vi "HTTPS Server Test with TCPIP Nodes.vi"() -> ()   [LabVIEW 2013]
uses:
  NI OpenSSL Socket/SSL_Lib/SSL-Lib/Library Paths.ctl
  NI OpenSSL Socket/SSL_Lib/SSL/SSL_Mode.ctl
  NI OpenSSL Socket/SSL_Lib/SSL-Lib/SSL-Lib.lvclass
  NI OpenSSL Socket/SSL_Lib/SSL-Context/SSL-Context.lvclass
  NI OpenSSL Socket/SSL_Lib/SSL/SSL.lvclass
panel:
  in  "stop":bool
  out "Read bytes":string
  out "Numeric":i32
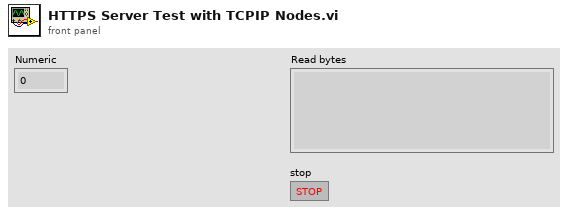
[diagram p1: front panel]
types:
  T1 = typedef "OpenSSL Socket.lvlib/SSL.lvclass/SSL_Mode.ctl" = i32
  T2 = typedef "OpenSSL Socket.lvlib/SSL-Lib.lvclass/Library Paths.ctl" = cluster{"SSL Library Path":path, "Crypto Library Path":path}
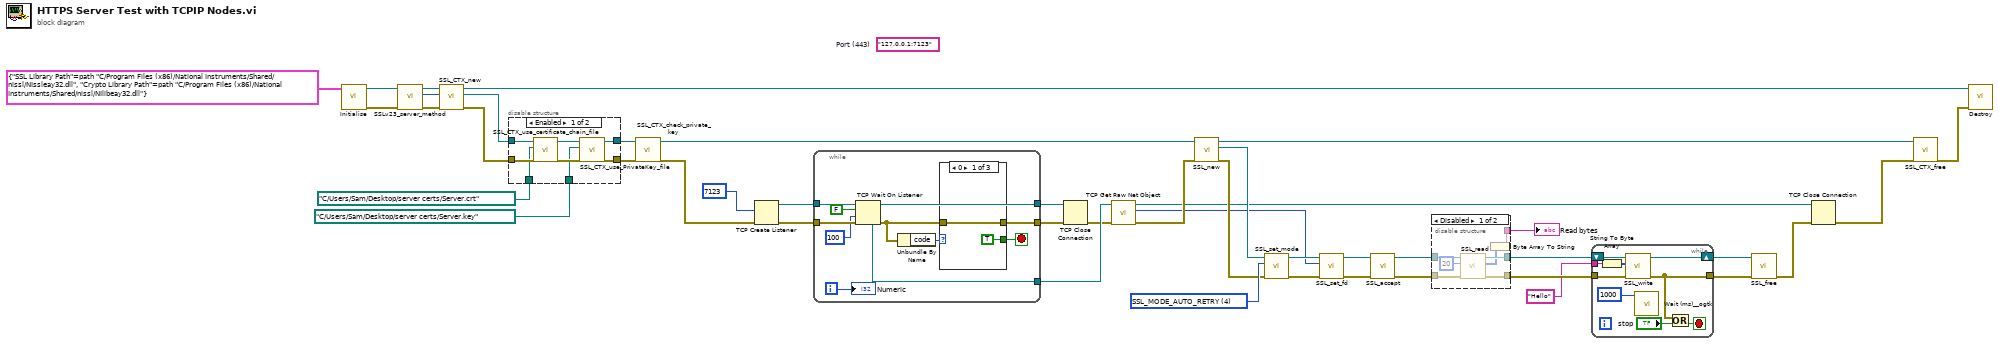
[diagram p0: block diagram]
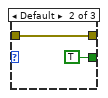
[diagram p3: hidden frame]
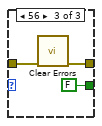
[diagram p4: hidden frame]
diagram:
  (unwired) "127.0.0.1:7123"  # Port (443)
  w31 = T1 4 items=["None"=0, "SSL_MODE_ENABLE_PARTIAL_WRITE"=1, "SSL_MODE_ACCEPT_MOVING_WRITE_BUFFER"=2, "SSL_MODE_AUTO_RETRY"=4, "SSL_MODE_RELEASE_BUFFERS"=16, "SSL_MODE_SEND_FALLBACK_SCSV"=128] ("Mode")
  n1 = call "Initialise.vi"("Library Paths"=T2 {"SSL Library Path"=path "C:/Program Files (x86)/National Instruments/Shared/nissl/NIssleay32.dll", "Crypto Library Path"=path "C:/Program Files (x86)/National Instruments/Shared/nissl/NIlibeay32.dll"}) -> ("error out"=w40:errorcluster, "SSL-Lib out"=w44:refnum<class "SSL-Lib.lvclass">)  [unwired: 9 in]
  n2 = call "SSLv23_server_method.vi"("error in (no error)"=w40, "SSL-Lib in"=w44) -> ("error out"=w38:errorcluster, "*SSL_Method"=w43:u64, "SSL-Lib out"=w42:refnum<class "SSL-Lib.lvclass">)  [unwired: 7 in]
  n3 = call "SSL_CTX_new.vi"("error in (no error)"=w38, "*SSL_Method"=w43, "SSL-Lib in"=w42) -> ("error out"=w37:errorcluster, "SSL-Context out"=w36:refnum<class "SSL-Context.lvclass">, "SSL-Lib out"=w30:refnum<class "SSL-Lib.lvclass">)  [unwired: 6 in]
  n4 = disable-structure shown="Enabled" {
    disable-tunnel: w37 -> [w50 w53]
    disable-tunnel: w36 -> [w49 w54]
    disable-tunnel: [w48 w53] -> w35
    disable-tunnel: [w47 w54] -> w34
    disable-tunnel: path "C:/Users/Sam/Desktop/server certs/Server.crt" -> [w46 _]
    disable-tunnel: path "C:/Users/Sam/Desktop/server certs/Server.key" -> [w45 _]
    frame Enabled {
      n5 = call "SSL_CTX_use_certificate_chain_file.vi"("error in (no error)"=w50, "Certificate Chain File"=w46, "SSL-Context in"=w49) -> ("error out"=w52:errorcluster, "SSL-Context out"=w51:refnum<class "SSL-Context.lvclass">)  [unwired: 7 in]
      n6 = call "SSL_CTX_use_PrivateKey_file.vi"("error in (no error)"=w52, "PrivateKey File"=w45, "SSL-Context in"=w51) -> ("error out"=w48:errorcluster, "SSL-Context out"=w47:refnum<class "SSL-Context.lvclass">)  [unwired: 7 in]
    }
    frame Disabled {
    }
  }
  n7 = call "SSL_CTX_check_private_key.vi"("error in (no error)"=w35, "SSL-Context in"=w34) -> ("error out"=w21:errorcluster, "SSL-Context out"=w20:refnum<class "SSL-Context.lvclass">)  [unwired: 8 in]
  n8 = TCP Create Listener(8:w21, 10:u16 7123 ("port")) -> (0:w28:errorcluster, 3:w27:refnum<k5>)  [unwired: 3 in, 1 out]
  n9 = while {
    tunnel: w28 -> [w65]
    tunnel: w27 -> [w64]
    tunnel: [w63] -> w26
    tunnel: [w59] -> w25
    tunnel: [w62] -> w24
    i -> [w55]
    stop <- w58 stop-if-true
    n10 = TCP Wait On Listener(8:w65, 9:100 ("timeout ms (wait forever: -1)"), 10:FALSE ("resolve remote address (T)"), 11:w64) -> (0:w60:errorcluster, 3:w63:refnum<k5>, 4:w62:refnum<k5>)  [unwired: 2 out]
    n11 = Unbundle By Name(w60) -> ("code"=w61:i32)
    n12 = case shown="0" w61 {
      tunnel: w60 -> [w67 w69 w72]
      tunnel: [w67 w69 w71] -> w59
      tunnel: [TRUE TRUE FALSE] -> w58
      frame 0 {
      }
      frame Default {
      }
      frame 56 {
        n13 = call <vilib>:"Clear Errors.vi"("error in (no error)"=w72) -> ("error out"=w71:errorcluster)  [unwired: 6 in]
      }
    }
    "Numeric" <- w55
  }
  n14 = TCP Close Connection(connection ID=w26, error in (no error)=w25) -> (error out=w23:errorcluster)  [unwired: 1 in, 1 out]
  n15 = call <vilib>:"TCP Get Raw Net Object.vi"("error in (no error)"=w23, "connection ID"=w24) -> ("error out"=w19:errorcluster, "raw net object"=w14:u64, "connection ID out"=w13:refnum<k5>)  [unwired: 7 in]
  n16 = call "SSL_new.vi"("error in (no error)"=w19, "SSL-Context in"=w20) -> ("error out"=w18:errorcluster, "SSL out"=w17:refnum<class "SSL.lvclass">, "SSL-Context out"=w12:refnum<class "SSL-Context.lvclass">)  [unwired: 7 in]
  n17 = call "SSL_set_mode.vi"("error in (no error)"=w18, "Mode"=w31, "SSL in"=w17) -> ("error out"=w15:errorcluster, "SSL out"=w16:refnum<class "SSL.lvclass">)  [unwired: 7 in]
  n18 = call "SSL_set_fd.vi"("error in (no error)"=w15, "fd"=w14, "SSL in"=w16) -> ("error out"=w11:errorcluster, "SSL out"=w10:refnum<class "SSL.lvclass">)  [unwired: 7 in]
  n19 = call "SSL_accept.vi"("error in (no error)"=w11, "SSL in"=w10) -> ("error out"=w8:errorcluster, "SSL out"=w7:refnum<class "SSL.lvclass">)  [unwired: 8 in]
  n20 = disable-structure shown="Disabled" {
    disable-tunnel: w8 -> [w79 w80]
    disable-tunnel: w7 -> [w78 w81]
    disable-tunnel: [w76 w81] -> w2
    disable-tunnel: [w75 w80] -> w3
    disable-tunnel: [w73 _] -> w6
    frame Disabled {
      n21 = call "SSL_read.vi"("error in (no error)"=w79, "Bytes to read"=20, "SSL in"=w78) -> ("error out"=w75:errorcluster, "Read bytes"=w74:u8[], "SSL out"=w76:refnum<class "SSL.lvclass">)  [unwired: 6 in]
      n22 = Byte Array To String(unsigned byte array=w74) -> (string=w73:string)
    }
    frame Enabled {
    }
  }
  "Read bytes" <- w6
  n23 = while {
    tunnel: w3 -> [w85]
    tunnel: [w83] -> w5
    shift-right: [w88] -> w4
    shift-left: w2 -> [w87]
    tunnel: "Hello" ("Write string") -> [w86]
    stop <- w84 stop-if-true
    n24 = String To Byte Array(string=w86) -> (unsigned byte array=w82:u8[])
    n25 = call "SSL_write.vi"("error in (no error)"=w85, "Write string"=w82, "SSL in"=w87) -> ("error out"=w83:errorcluster, "SSL out"=w88:refnum<class "SSL.lvclass">)  [unwired: 6 in, 1 out]
    n26 = call <userlib>:"Wait (ms)__ogtk.vi"("milliseconds to wait"=u32 1000) -> ()  [unwired: 9 in, 2 out]
    n27 = Or(x=w83, y="stop") -> (x .or. y?=w84:bool)
  }
  n28 = call "SSL_free.vi"("error in (no error)"=w5, "SSL in"=w4) -> ("error out"=w9:errorcluster)  [unwired: 9 in]
  n29 = TCP Close Connection(connection ID=w13, error in (no error)=w9) -> (error out=w22:errorcluster)  [unwired: 1 in, 1 out]
  n30 = call "SSL_CTX_free.vi"("error in (no error)"=w22, "SSL-Context in"=w12) -> ("error out"=w39:errorcluster)  [unwired: 9 in]
  n31 = call "Destroy.vi"("error in (no error)"=w39, "SSL-Lib in"=w30) -> ()  [unwired: 9 in, 1 out]
